vi "Cycle_Diag_Table_Read_Mio.vi"(7 "ERD Data In":T2[](array[typedef]) {"ERD Number" format="%.0x"}, 11 "error in (no error)":errorcluster) -> (2 "Cycle Buffer Status":T1, 3 "Diag Cycle String Out":string[][](array[string]), 15 "error out (no error)":errorcluster)   [LabVIEW 2021]
uses:
  Common/LabVIEW GEA2 Toolkit/GEA3/type defs/ERD Read Data Out.ctl
  type defs/Cycle_Diag_Buffer_Status.ctl
panel:
  out "length":i32
  out "Data":string
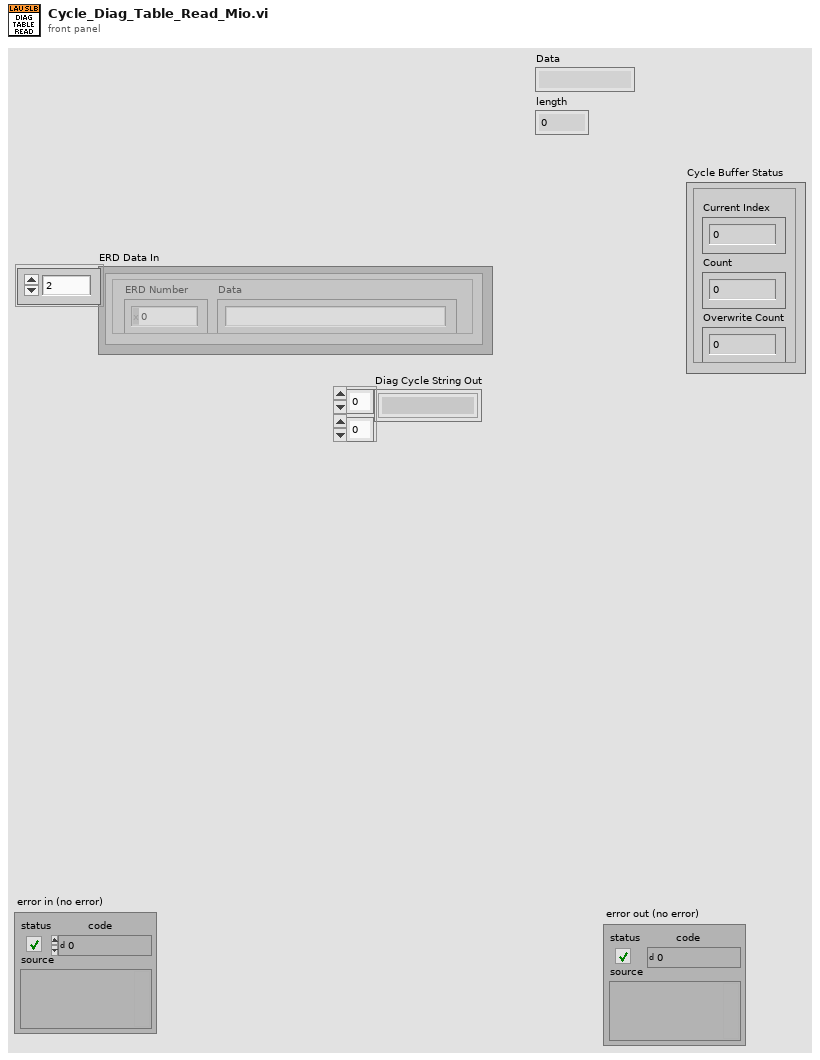
[diagram p1: front panel]
types:
  T1 = typedef "Cycle_Diag_Buffer_Status.ctl" = cluster{"Current Index":u16, "Count":u16, "Overwrite Count":u16}
  T2 = typedef "ERD Read Data Out.ctl" = cluster{"ERD Number":u16, "Data":string}
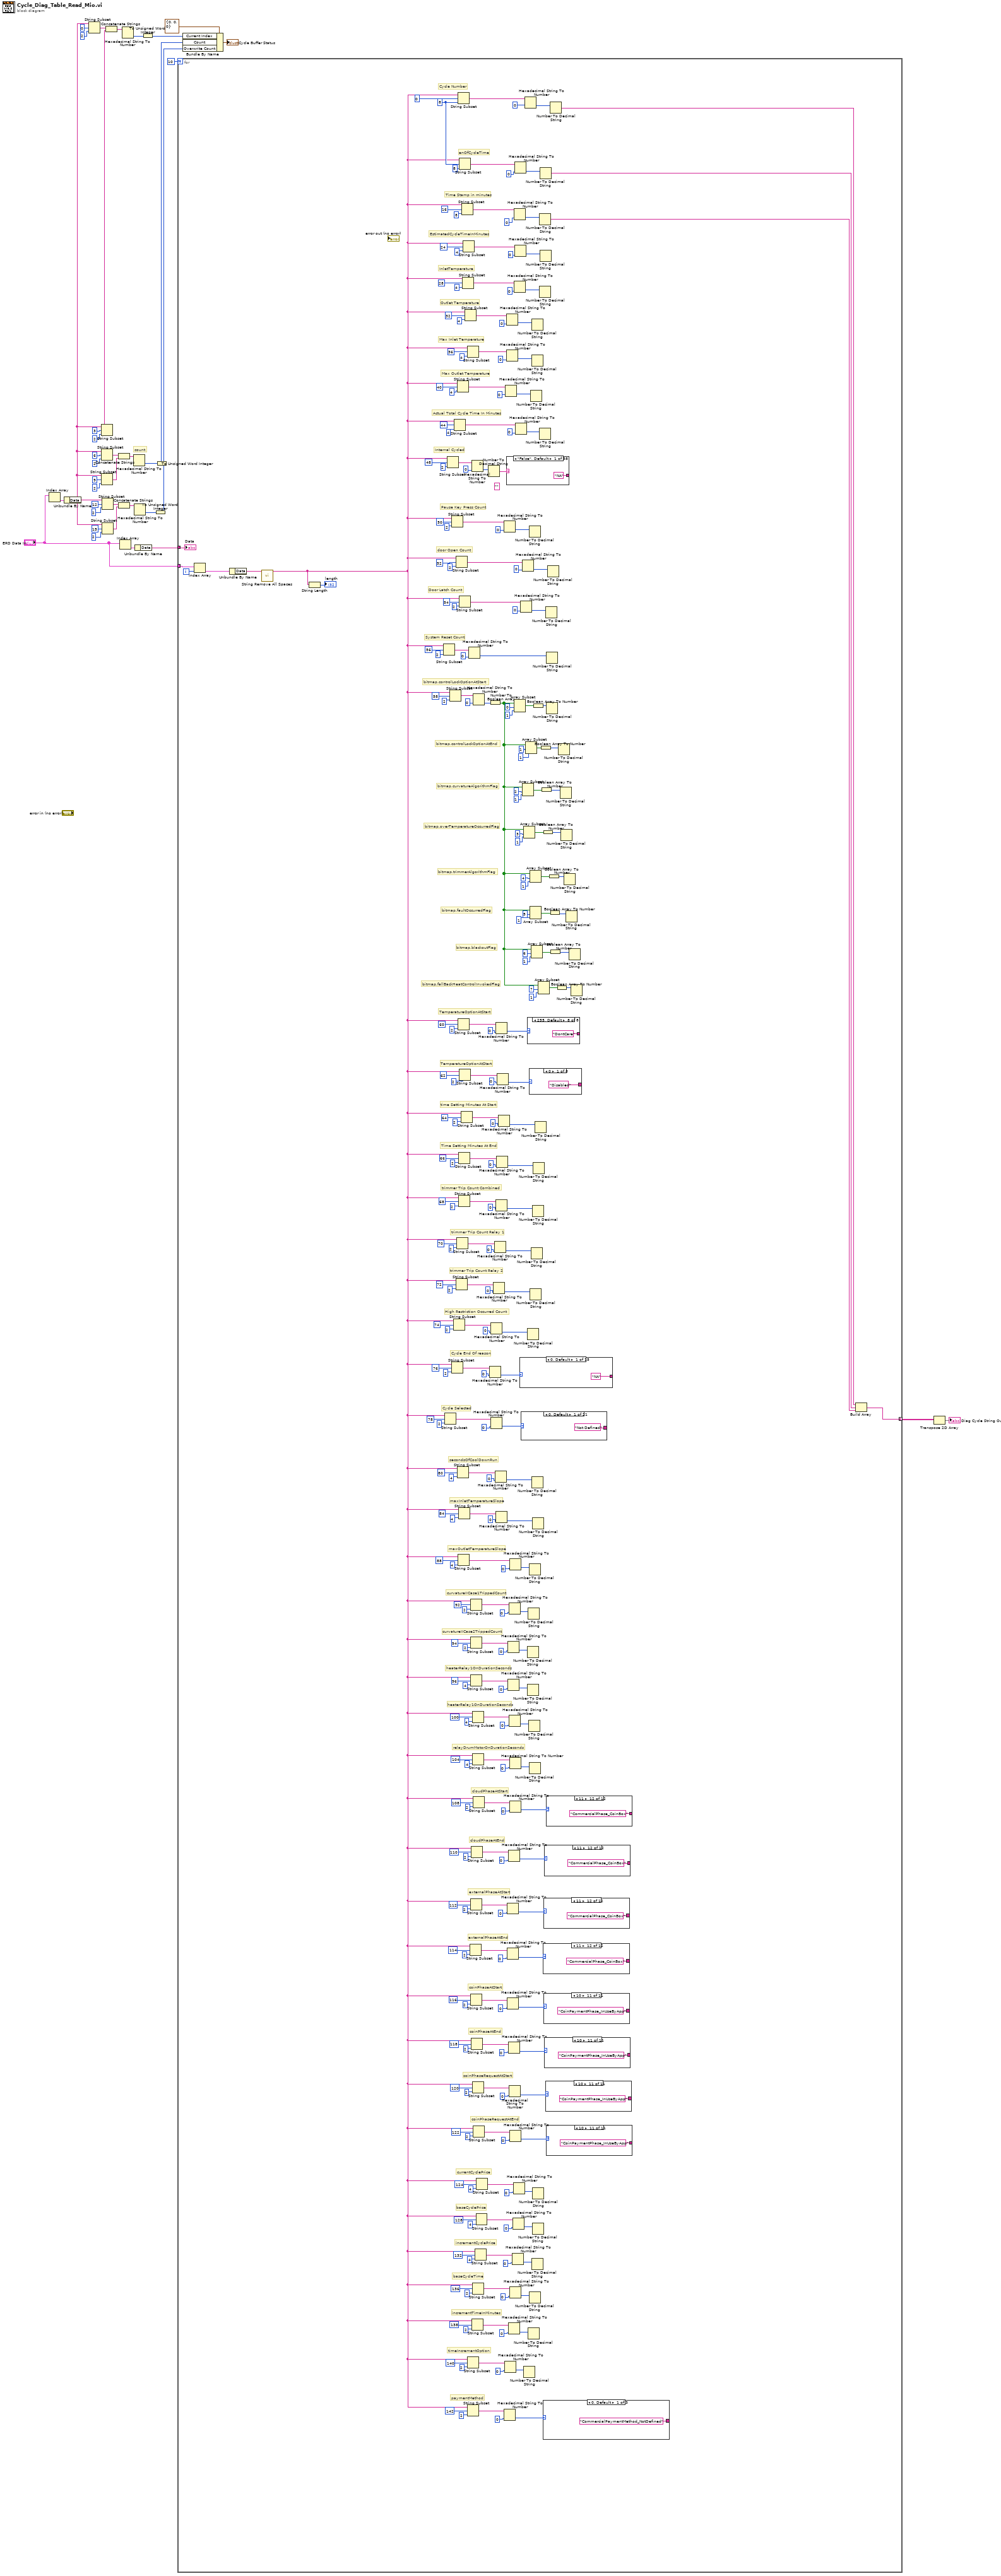
[diagram p0: block diagram]
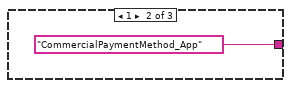
[diagram p2: hidden frame]
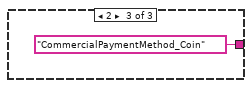
[diagram p3: hidden frame]
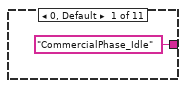
[diagram p4: hidden frame]
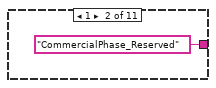
[diagram p5: hidden frame]
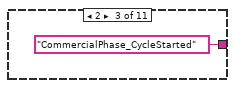
[diagram p6: hidden frame]
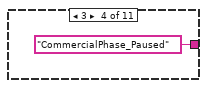
[diagram p7: hidden frame]
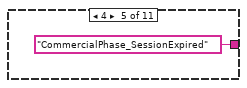
[diagram p8: hidden frame]
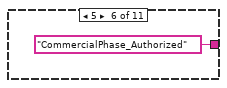
[diagram p9: hidden frame]
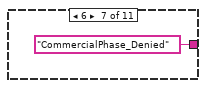
[diagram p10: hidden frame]
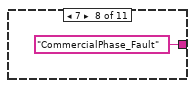
[diagram p11: hidden frame]
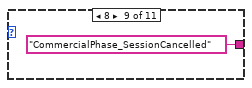
[diagram p12: hidden frame]
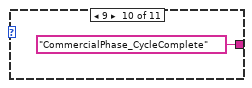
[diagram p13: hidden frame]
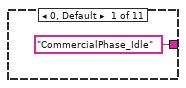
[diagram p14: hidden frame]
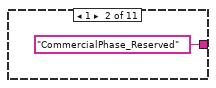
[diagram p15: hidden frame]
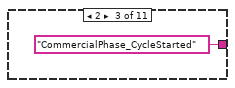
[diagram p16: hidden frame]
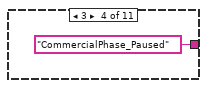
[diagram p17: hidden frame]
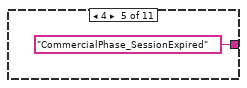
[diagram p18: hidden frame]
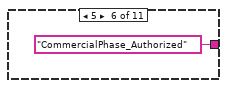
[diagram p19: hidden frame]
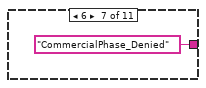
[diagram p20: hidden frame]
diagram:
  # "count"
  n1 = Index Array(array="ERD Data In") -> (element=w30:T2)  [unwired: 1 in]
  n2 = Unbundle By Name(w30) -> ("Data"=w10:string)
  n3 = String Subset(string=w10, offset (0)=0, length (rest)=2 ("length (rest)")) -> (substring=w19:string)
  n4 = String Subset(string=w10, offset (0)=3, length (rest)=2 ("length (rest)")) -> (substring=w20:string)
  n5 = String Subset(string=w10, offset (0)=6, length (rest)=2 ("length (rest)")) -> (substring=w34:string)
  n6 = String Subset(string=w10, offset (0)=9, length (rest)=2 ("length (rest)")) -> (substring=w33:string)
  n7 = String Subset(string=w10, offset (0)=12, length (rest)=2 ("length (rest)")) -> (substring=w21:string)
  n8 = String Subset(string=w10, offset (0)=15, length (rest)=2 ("length (rest)")) -> (substring=w22:string)
  n9 = Concatenate Strings(w19, w20) -> (w23:string)
  n10 = Concatenate Strings(w34, w33) -> (w32:string)
  n11 = Concatenate Strings(w21, w22) -> (w24:string)
  n12 = Index Array(array="ERD Data In") -> (element=w5:T2)  [unwired: 1 in]
  n13 = Hexadecimal String To Number(string=w23) -> (number=w25:u32)  [unwired: 2 in, 1 out]
  n14 = Hexadecimal String To Number(string=w32) -> (number=w31:u32)  [unwired: 2 in, 1 out]
  n15 = Hexadecimal String To Number(string=w24) -> (number=w26:u32)  [unwired: 2 in, 1 out]
  n16 = Unbundle By Name(w5) -> ("Data"=w4:string)
  n17 = To Unsigned Word Integer(number=w25) -> (unsigned 16bit integer=w27:u16)
  n18 = To Unsigned Word Integer(number=w26) -> (unsigned 16bit integer=w28:u16)
  n19 = To Unsigned Word Integer(number=w31) -> (unsigned 16bit integer=w2:u16)
  n20 = for {
    N: 10 -> [_]
    tunnel: [w48] -> w7 mode=indexing
    tunnel: w4 -> [w42]
    tunnel: "ERD Data In" -> [w44]
    i -> [w43]
    (unwired) ""
    w261 = 8 ("length (rest)")
    # "paymentMethod"
    # "timeIncrementOption"
    # "incrementTimeInMinutes"
    # "baseCycleTime"
    # "incrementCyclePrice"
    # "baseCyclePrice"
    # "currentCyclePrice"
    # "coinPhaseRequestAtEnd"
    # "coinPhaseRequestAtStart"
    # "coinPhaseAtEnd"
    # "coinPhaseAtStart"
    # "externalPhaseAtEnd"
    # "externalPhaseAtStart"
    # "cloudPhaseAtEnd"
    # "cloudPhaseAtStart"
    # "relayDrumMotorOnDurationSeconds"
    # "heaterRelay1OnDurationSeconds"
    # "heaterRelay1OnDurationSeconds"
    # "maxInletTemperatureSlope"
    # "secondsOfCoolDownRun"
    # "Cycle End Of reason"
    # "High Restriction Occurred Count"
    # "trimmer Trip Count Relay 2"
    # "trimmer Trip Count Relay 1"
    # "trimmer Trip Count Combined"
    # "Time Setting Minutes At End"
    # "time Setting Minutes At Start"
    # "TemperatureOptionAtStart"
    # "TemperatureOptionAtStart"
    # "bitmap.overTemperatureOccurredFlag"
    # "bitmap.curvatureAlgorithmFlag"
    # "bitmap.controlLockOptionAtEnd"
    # "Pause Key Press Count"
    # "InletTemperature"
    # "curvatureIICase1TrippedCount"
    # "curvatureIICase2TrippedCount"
    # "maxOutletTemperatureSlope"
    # "Cycle Selected"
    # "bitmap.fallBackHeatControlInvokedFlag"
    # "bitmap.blackoutFlag"
    # "bitmap.faultOccurredFlag"
    # "bitmap.trimmerAlgorithmFlag"
    # "bitmap.controlLockOptionAtStart"
    # "System Reset Count"
    # "Door Latch Count"
    # "door Open Count"
    # "Internal Cycled"
    # "Actual Total Cycle Time In Minutes"
    # "Max Outlet Temperature"
    # "Max Inlet Temperature"
    # "Outlet Temperature"
    # "EstimatedCycleTimeInMinutes"
    # "Time Stamp in minutes"
    # "enOfCycleTime"
    # "Cycle Number"
    n21 = Index Array(array=w44, index=w43) -> (element=w41:T2)
    n22 = Unbundle By Name(w41) -> ("Data"=w39:string)
    n23 = call "String Remove All Spaces.vi"("Input String"=w39) -> ("Spaces Removed"=w38:string)  [unwired: 13 in, 1 out]
    n24 = String Length(string=w38) -> (length=→"length":i32)
    n25 = String Subset(string=w38, offset (0)=56, length (rest)=2 ("length (rest)")) -> (substring=w235:string)
    n26 = String Subset(string=w38, offset (0)=78, length (rest)=2 ("length (rest)")) -> (substring=w272:string)
    n27 = String Subset(string=w38, offset (0)=48, length (rest)=2 ("length (rest)")) -> (substring=w245:string)
    n28 = String Subset(string=w38, offset (0)=58, length (rest)=2 ("length (rest)")) -> (substring=w234:string)
    n29 = String Subset(string=w38, offset (0)=50, length (rest)=2 ("length (rest)")) -> (substring=w242:string)
    n30 = String Subset(string=w38, offset (0)=76, length (rest)=2 ("length (rest)")) -> (substring=w192:string)
    n31 = String Subset(string=w38, offset (0)=74, length (rest)=2 ("length (rest)")) -> (substring=w193:string)
    n32 = String Subset(string=w38, offset (0)=44, length (rest)=4 ("length (rest)")) -> (substring=w247:string)
    n33 = String Subset(string=w38, offset (0)=72, length (rest)=2 ("length (rest)")) -> (substring=w200:string)
    n34 = String Subset(string=w38, offset (0)=52, length (rest)=2 ("length (rest)")) -> (substring=w240:string)
    n35 = String Subset(string=w38, offset (0)=70, length (rest)=2 ("length (rest)")) -> (substring=w205:string)
    n36 = String Subset(string=w38, offset (0)=40, length (rest)=4 ("length (rest)")) -> (substring=w249:string)
    n37 = String Subset(string=w38, offset (0)=80, length (rest)=4 ("length (rest)")) -> (substring=w181:string)
    n38 = String Subset(string=w38, offset (0)=0, length (rest)=w261) -> (substring=w262:string)
    n39 = String Subset(string=w38, offset (0)=60, length (rest)=2 ("length (rest)")) -> (substring=w231:string)
    n40 = String Subset(string=w38, offset (0)=88, length (rest)=4 ("length (rest)")) -> (substring=w269:string)
    n41 = String Subset(string=w38, offset (0)=68, length (rest)=2 ("length (rest)")) -> (substring=w210:string)
    n42 = String Subset(string=w38, offset (0)=84, length (rest)=4 ("length (rest)")) -> (substring=w180:string)
    n43 = String Subset(string=w38, offset (0)=66, length (rest)=2 ("length (rest)")) -> (substring=w215:string)
    n44 = String Subset(string=w38, offset (0)=w261, length (rest)=8 ("length (rest)")) -> (substring=w260:string)
    n45 = String Subset(string=w38, offset (0)=54, length (rest)=2 ("length (rest)")) -> (substring=w238:string)
    n46 = String Subset(string=w38, offset (0)=62, length (rest)=2 ("length (rest)")) -> (substring=w224:string)
    n47 = String Subset(string=w38, offset (0)=64, length (rest)=2 ("length (rest)")) -> (substring=w220:string)
    n48 = String Subset(string=w38, offset (0)=16, length (rest)=8 ("length (rest)")) -> (substring=w259:string)
    n49 = String Subset(string=w38, offset (0)=28, length (rest)=4 ("length (rest)")) -> (substring=w255:string)
    n50 = String Subset(string=w38, offset (0)=24, length (rest)=4 ("length (rest)")) -> (substring=w257:string)
    n51 = String Subset(string=w38, offset (0)=32, length (rest)=4 ("length (rest)")) -> (substring=w253:string)
    n52 = String Subset(string=w38, offset (0)=36, length (rest)=4 ("length (rest)")) -> (substring=w251:string)
    n53 = String Subset(string=w38, offset (0)=142, length (rest)=2 ("length (rest)")) -> (substring=w85:string)
    n54 = String Subset(string=w38, offset (0)=140, length (rest)=2 ("length (rest)")) -> (substring=w89:string)
    n55 = Hexadecimal String To Number(string=w235, default (0uL)=u16 0) -> (number=w276:u16)  [unwired: 1 in, 1 out]
    n56 = String Subset(string=w38, offset (0)=114, length (rest)=2 ("length (rest)")) -> (substring=w140:string)
    n57 = String Subset(string=w38, offset (0)=92, length (rest)=2 ("length (rest)")) -> (substring=w266:string)
    n58 = String Subset(string=w38, offset (0)=112, length (rest)=2 ("length (rest)")) -> (substring=w145:string)
    n59 = String Subset(string=w38, offset (0)=116, length (rest)=2 ("length (rest)")) -> (substring=w135:string)
    n60 = String Subset(string=w38, offset (0)=94, length (rest)=2 ("length (rest)")) -> (substring=w263:string)
    n61 = String Subset(string=w38, offset (0)=96, length (rest)=4 ("length (rest)")) -> (substring=w171:string)
    n62 = String Subset(string=w38, offset (0)=110, length (rest)=2 ("length (rest)")) -> (substring=w150:string)
    n63 = String Subset(string=w38, offset (0)=118, length (rest)=2 ("length (rest)")) -> (substring=w130:string)
    n64 = Hexadecimal String To Number(string=w245, default (0uL)=u32 0) -> (number=w284:u32)  [unwired: 1 in, 1 out]
    n65 = String Subset(string=w38, offset (0)=138, length (rest)=2 ("length (rest)")) -> (substring=w94:string)
    n66 = String Subset(string=w38, offset (0)=100, length (rest)=4 ("length (rest)")) -> (substring=w164:string)
    n67 = String Subset(string=w38, offset (0)=120, length (rest)=2 ("length (rest)")) -> (substring=w120:string)
    n68 = String Subset(string=w38, offset (0)=104, length (rest)=4 ("length (rest)")) -> (substring=w161:string)
    n69 = String Subset(string=w38, offset (0)=136, length (rest)=2 ("length (rest)")) -> (substring=w101:string)
    n70 = Hexadecimal String To Number(string=w234, default (0uL)=u16 0) -> (number=w79:u16)  [unwired: 1 in, 1 out]
    n71 = String Subset(string=w38, offset (0)=108, length (rest)=2 ("length (rest)")) -> (substring=w155:string)
    n72 = String Subset(string=w38, offset (0)=122, length (rest)=2 ("length (rest)")) -> (substring=w125:string)
    n73 = String Subset(string=w38, offset (0)=132, length (rest)=4 ("length (rest)")) -> (substring=w106:string)
    n74 = String Subset(string=w38, offset (0)=128, length (rest)=4 ("length (rest)")) -> (substring=w109:string)
    n75 = String Subset(string=w38, offset (0)=124, length (rest)=4 ("length (rest)")) -> (substring=w116:string)
    n76 = Number To Decimal String(number=w284) -> (decimal integer string=w243:string)  [unwired: 1 in]
    n77 = Hexadecimal String To Number(string=w192, default (0uL)=u8 0) -> (number=w188:u8)  [unwired: 1 in, 1 out]
    n78 = Number To Boolean Array(number=w79) -> (Boolean array=w49:bool[])
    n79 = Hexadecimal String To Number(string=w272, default (0uL)=u32 0) -> (number=w186:u32)  [unwired: 1 in, 1 out]
    n80 = Hexadecimal String To Number(string=w193, default (0uL)=u32 0) -> (number=w197:u32)  [unwired: 1 in, 1 out]
    n81 = Hexadecimal String To Number(string=w200, default (0uL)=u8 0) -> (number=w198:u8)  [unwired: 1 in, 1 out]
    n82 = Hexadecimal String To Number(string=w205, default (0uL)=u32 0) -> (number=w207:u32)  [unwired: 1 in, 1 out]
    n83 = Hexadecimal String To Number(string=w181, default (0uL)=u32 0) -> (number=w185:u32)  [unwired: 1 in, 1 out]
    n84 = Hexadecimal String To Number(string=w231, default (0uL)=u32 0) -> (number=w228:u32)  [unwired: 1 in, 1 out]
    n85 = Hexadecimal String To Number(string=w210, default (0uL)=u32 0) -> (number=w208:u32)  [unwired: 1 in, 1 out]
    n86 = Hexadecimal String To Number(string=w180, default (0uL)=u8 0) -> (number=w176:u8)  [unwired: 1 in, 1 out]
    n87 = Hexadecimal String To Number(string=w215, default (0uL)=u32 0) -> (number=w217:u32)  [unwired: 1 in, 1 out]
    n88 = Hexadecimal String To Number(string=w224, default (0uL)=u32 0) -> (number=w227:u32)  [unwired: 1 in, 1 out]
    n89 = Hexadecimal String To Number(string=w220, default (0uL)=u32 0) -> (number=w218:u32)  [unwired: 1 in, 1 out]
    n90 = Hexadecimal String To Number(string=w242, default (0uL)=u16 0) -> (number=w281:u16)  [unwired: 1 in, 1 out]
    n91 = Hexadecimal String To Number(string=w85, default (0uL)=u8 0) -> (number=w83:u8)  [unwired: 1 in, 1 out]
    n92 = Hexadecimal String To Number(string=w89, default (0uL)=u8 0) -> (number=w90:u8)  [unwired: 1 in, 1 out]
    n93 = Hexadecimal String To Number(string=w249, default (0uL)=u32 0) -> (number=w288:u32)  [unwired: 1 in, 1 out]
    n94 = Hexadecimal String To Number(string=w253, default (0uL)=u32 0) -> (number=w292:u32)  [unwired: 1 in, 1 out]
    n95 = Hexadecimal String To Number(string=w251, default (0uL)=u32 0) -> (number=w289:u32)  [unwired: 1 in, 1 out]
    n96 = case shown="\"False\", Default" w243 {
      tunnel: ["NA" "Unmapped" "MixedLoad" "Casuals" "Delicates" "SpeedDry" "Jeans" "TimedDry" "WarmUp" "AirFluff" "SteamDewrinkle" "SteamRefresh" "SanitizeDry" "BulkyItems" "TowelsSheets" "Cottons" "CasualsLessDry" "CasualsMoreDry" "CottonsLessDry" "CottonsOptimumDry" "CottonsMoreDry" "DelicatesLessDry" "DelicatesMoreDry" "TimedDry1" "TimedDry2" "TimedDry3" "TimedDry4" "TimedDry5" "TimedDry6" "ActiveWear" "DeWrinkle" "EnergySaver" "WasherLink" "BlockedVent" "SmartVent" "Scent" "Max" "Downloaded"] -> _
      frame "False", Default {
      }
      frame "0" {
      }
      frame "1" {
      }
      frame "2" {
      }
      frame "3" {
      }
      frame "4" {
      }
      frame "5" {
      }
      frame "6" {
      }
      frame "7" {
      }
      frame "8" {
      }
      frame "9" {
      }
      frame "10" {
      }
      frame "11" {
      }
      frame "12" {
      }
      frame "13" {
      }
      frame "14" {
      }
      frame "15" {
      }
      frame "16" {
      }
      frame "17" {
      }
      frame "18" {
      }
      frame "19" {
      }
      frame "20" {
      }
      frame "21" {
      }
      frame "22" {
      }
      frame "23" {
      }
      frame "24" {
      }
      frame "25" {
      }
      frame "26" {
      }
      frame "27" {
      }
      frame "28" {
      }
      frame "29" {
      }
      frame "30" {
      }
      frame "31" {
      }
      frame "32" {
      }
      frame "33" {
      }
      frame "34" {
      }
      frame "35" {
      }
      frame "36" {
      }
    }
    n97 = Hexadecimal String To Number(string=w140, default (0uL)=u8 0) -> (number=w142:u8)  [unwired: 1 in, 1 out]
    n98 = Hexadecimal String To Number(string=w145, default (0uL)=u8 0) -> (number=w143:u8)  [unwired: 1 in, 1 out]
    n99 = Hexadecimal String To Number(string=w135, default (0uL)=u8 0) -> (number=w133:u8)  [unwired: 1 in, 1 out]
    n100 = Hexadecimal String To Number(string=w263, default (0uL)=u32 0) -> (number=w264:u32)  [unwired: 1 in, 1 out]
    n101 = Hexadecimal String To Number(string=w171, default (0uL)=u32 0) -> (number=w170:u32)  [unwired: 1 in, 1 out]
    n102 = Hexadecimal String To Number(string=w150, default (0uL)=u8 0) -> (number=w152:u8)  [unwired: 1 in, 1 out]
    n103 = Hexadecimal String To Number(string=w130, default (0uL)=u8 0) -> (number=w132:u8)  [unwired: 1 in, 1 out]
    n104 = Hexadecimal String To Number(string=w94, default (0uL)=u32 0) -> (number=w95:u32)  [unwired: 1 in, 1 out]
    n105 = Hexadecimal String To Number(string=w266, default (0uL)=u32 0) -> (number=w268:u32)  [unwired: 1 in, 1 out]
    n106 = Hexadecimal String To Number(string=w164, default (0uL)=u32 0) -> (number=w165:u32)  [unwired: 1 in, 1 out]
    n107 = Hexadecimal String To Number(string=w120, default (0uL)=u8 0) -> (number=w122:u8)  [unwired: 1 in, 1 out]
    n108 = Hexadecimal String To Number(string=w161, default (0uL)=u32 0) -> (number=w160:u32)  [unwired: 1 in, 1 out]
    n109 = Hexadecimal String To Number(string=w101, default (0uL)=u8 0) -> (number=w100:u8)  [unwired: 1 in, 1 out]
    n110 = Hexadecimal String To Number(string=w269, default (0uL)=u32 0) -> (number=w270:u32)  [unwired: 1 in, 1 out]
    n111 = Hexadecimal String To Number(string=w155, default (0uL)=u8 0) -> (number=w153:u8)  [unwired: 1 in, 1 out]
    n112 = Hexadecimal String To Number(string=w125, default (0uL)=u8 0) -> (number=w123:u8)  [unwired: 1 in, 1 out]
    n113 = Hexadecimal String To Number(string=w106, default (0uL)=u32 0) -> (number=w105:u32)  [unwired: 1 in, 1 out]
    n114 = Hexadecimal String To Number(string=w109, default (0uL)=u32 0) -> (number=w110:u32)  [unwired: 1 in, 1 out]
    n115 = Hexadecimal String To Number(string=w116, default (0uL)=u32 0) -> (number=w115:u32)  [unwired: 1 in, 1 out]
    n116 = Array Subset(array=w49, index=0, length=1) -> (w80:bool[])
    n117 = Hexadecimal String To Number(string=w259, default (0uL)=u32 0) -> (number=w300:u32)  [unwired: 1 in, 1 out]
    n118 = Hexadecimal String To Number(string=w255, default (0uL)=u32 0) -> (number=w293:u32)  [unwired: 1 in, 1 out]
    n119 = Hexadecimal String To Number(string=w260, default (0uL)=u32 0) -> (number=w301:u32)  [unwired: 1 in, 1 out]
    n120 = Hexadecimal String To Number(string=w257, default (0uL)=u32 0) -> (number=w299:u32)  [unwired: 1 in, 1 out]
    n121 = Hexadecimal String To Number(string=w247, default (0uL)=u32 0) -> (number=w285:u32)  [unwired: 1 in, 1 out]
    n122 = case shown="0, Default" w188 {
      tunnel: ["NA" "EmptyDrum" "DryLoad" "CoolDownPaused" "xtendedTumblePaused" "KnobChange" "PowerButtonPressed" "CycleComplete" "EventSequenceCommunicationIssue" "CriticalFault" "RemoteStop" "ExtremeHeatDetected" "NonPausableCyclePaused" "SafetyCriticalWatchdogTimeout" "DontCare"] -> _
      frame 0, Default {
      }
      frame 1 {
      }
      frame 2 {
      }
      frame 3 {
      }
      frame 4 {
      }
      frame 5 {
      }
      frame 6 {
      }
      frame 7 {
      }
      frame 8 {
      }
      frame 9 {
      }
      frame 10 {
      }
      frame 11 {
      }
      frame 12 {
      }
      frame 13 {
      }
      frame 14 {
      }
    }
    n123 = Hexadecimal String To Number(string=w238, default (0uL)=u16 0) -> (number=w277:u16)  [unwired: 1 in, 1 out]
    n124 = case shown="0, Default" w186 {
      tunnel: ["Not Defined" "Bulky Items" "Sanitize" "Towels/Sheets" "Mixed Load" "Jeans" "Delicates" "Cottons" "Easy Care" "Active Wear" "Timed Dry" "DeWrinkle" "Quick/Air Fluff" "Steam Refresh" "Steam Dewrinkle" "Speed Dry" "Mixed" "Quick dry" "Casuals" "Warm up" "Energy Saver"] -> _
      frame 0, Default {
      }
      frame 4 {
      }
      frame 5 {
      }
      frame 6 {
      }
      frame 8 {
      }
      frame 11 {
      }
      frame 13 {
      }
      frame 128 {
      }
      frame 129 {
      }
      frame 130 {
      }
      frame 131 {
      }
      frame 132 {
      }
      frame 133 {
      }
      frame 134 {
      }
      frame 135 {
      }
      frame 136 {
      }
      frame 137 {
      }
      frame 138 {
      }
      frame 139 {
      }
      frame 140 {
      }
      frame 141 {
      }
    }
    n125 = Hexadecimal String To Number(string=w240, default (0uL)=u16 0) -> (number=w280:u16)  [unwired: 1 in, 1 out]
    n126 = Array Subset(array=w49, index=2, length=1) -> (w71:bool[])
    n127 = Array Subset(array=w49, index=3, length=1) -> (w67:bool[])
    n128 = Number To Decimal String(number=w90) -> ()  [unwired: 1 in, 1 out]
    n129 = Hexadecimal String To Number(string=w262, default (0uL)=u32 0) -> (number=w302:u32)  [unwired: 1 in, 1 out]
    n130 = Array Subset(array=w49, index=1, length=1) -> (w75:bool[])
    n131 = Number To Decimal String(number=w264) -> ()  [unwired: 1 in, 1 out]
    n132 = Number To Decimal String(number=w170) -> ()  [unwired: 1 in, 1 out]
    n133 = case shown="255, Default" w228 {
      tunnel: ["Disabled" "NoHeat" "ExtraLow" "Low" "Medium" "High" "Max" "DontCare"] -> _
      frame 0 {
      }
      frame 1 {
      }
      frame 2 {
      }
      frame 3 {
      }
      frame 4 {
      }
      frame 5 {
      }
      frame 6 {
      }
      frame 255, Default {
      }
    }
    n134 = Number To Decimal String(number=w197) -> ()  [unwired: 1 in, 1 out]
    n135 = Number To Decimal String(number=w95) -> ()  [unwired: 1 in, 1 out]
    n136 = Number To Decimal String(number=w268) -> ()  [unwired: 1 in, 1 out]
    n137 = Number To Decimal String(number=w165) -> ()  [unwired: 1 in, 1 out]
    n138 = Number To Decimal String(number=w281) -> ()  [unwired: 1 in, 1 out]
    n139 = case shown="0" w227 {
      tunnel: ["Disabled" "NoHeat" "ExtraLow" "Low" "Medium" "High" "Max" "DontCare"] -> _
      frame 0 {
      }
      frame 1 {
      }
      frame 2 {
      }
      frame 3 {
      }
      frame 4 {
      }
      frame 5 {
      }
      frame 6 {
      }
      frame 255, Default {
      }
    }
    n140 = Number To Decimal String(number=w160) -> ()  [unwired: 1 in, 1 out]
    n141 = Number To Decimal String(number=w100) -> ()  [unwired: 1 in, 1 out]
    n142 = Number To Decimal String(number=w270) -> ()  [unwired: 1 in, 1 out]
    n143 = Array Subset(array=w49, index=4, length=1) -> (w63:bool[])
    n144 = Array Subset(array=w49, index=5, length=1) -> (w59:bool[])
    n145 = Number To Decimal String(number=w198) -> ()  [unwired: 1 in, 1 out]
    n146 = Number To Decimal String(number=w288) -> ()  [unwired: 1 in, 1 out]
    n147 = Array Subset(array=w49, index=6, length=1) -> (w55:bool[])
    n148 = Number To Decimal String(number=w207) -> ()  [unwired: 1 in, 1 out]
    n149 = Number To Decimal String(number=w292) -> ()  [unwired: 1 in, 1 out]
    n150 = Number To Decimal String(number=w289) -> ()  [unwired: 1 in, 1 out]
    n151 = Number To Decimal String(number=w185) -> ()  [unwired: 1 in, 1 out]
    n152 = Number To Decimal String(number=w105) -> ()  [unwired: 1 in, 1 out]
    n153 = Number To Decimal String(number=w110) -> ()  [unwired: 1 in, 1 out]
    n154 = Boolean Array To Number(Boolean array=w80) -> (number=w78:u32)
    n155 = Number To Decimal String(number=w208) -> ()  [unwired: 1 in, 1 out]
    n156 = Number To Decimal String(number=w176) -> ()  [unwired: 1 in, 1 out]
    n157 = Number To Decimal String(number=w115) -> ()  [unwired: 1 in, 1 out]
    n158 = Number To Decimal String(number=w217) -> ()  [unwired: 1 in, 1 out]
    n159 = Number To Decimal String(number=w218) -> ()  [unwired: 1 in, 1 out]
    n160 = Array Subset(array=w49, index=7, length=1) -> (w51:bool[])
    n161 = Number To Decimal String(number=w300) -> (decimal integer string=w45:string)  [unwired: 1 in]
    n162 = Number To Decimal String(number=w293) -> ()  [unwired: 1 in, 1 out]
    n163 = Number To Decimal String(number=w285) -> ()  [unwired: 1 in, 1 out]
    n164 = Number To Decimal String(number=w301) -> (decimal integer string=w46:string)  [unwired: 1 in]
    n165 = Number To Decimal String(number=w299) -> ()  [unwired: 1 in, 1 out]
    n166 = Boolean Array To Number(Boolean array=w75) -> (number=w74:u32)
    n167 = Boolean Array To Number(Boolean array=w71) -> (number=w70:u32)
    n168 = Boolean Array To Number(Boolean array=w67) -> (number=w66:u32)
    n169 = case shown="0, Default" w83 {
      tunnel: ["CommercialPaymentMethod_NotDefined" "CommercialPaymentMethod_App" "CommercialPaymentMethod_Coin"] -> _
      frame 0, Default {
      }
      frame 1 {
      }
      frame 2 {
      }
    }
    n170 = case shown="11" w142 {
      tunnel: ["CommercialPhase_Idle" "CommercialPhase_Reserved" "CommercialPhase_CycleRequested" "CommercialPhase_CycleStarted" "CommercialPhase_Paused" "CommercialPhase_SessionExpired" "CommercialPhase_Authorized" "CommercialPhase_Denied" "CommercialPhase_Fault" "CommercialPhase_SessionCancelled" "CommercialPhase_CycleComplete" "CommercialPhase_CoinBox"] -> _
      frame 0, Default {
      }
      frame 1 {
      }
      frame 2 {
      }
      frame 3 {
      }
      frame 4 {
      }
      frame 5 {
      }
      frame 6 {
      }
      frame 7 {
      }
      frame 8 {
      }
      frame 9 {
      }
      frame 10 {
      }
      frame 11 {
      }
    }
    n171 = case shown="11" w143 {
      tunnel: ["CommercialPhase_Idle" "CommercialPhase_Reserved" "CommercialPhase_CycleRequested" "CommercialPhase_CycleStarted" "CommercialPhase_Paused" "CommercialPhase_SessionExpired" "CommercialPhase_Authorized" "CommercialPhase_Denied" "CommercialPhase_Fault" "CommercialPhase_SessionCancelled" "CommercialPhase_CycleComplete" "CommercialPhase_CoinBox"] -> _
      frame 0, Default {
      }
      frame 1 {
      }
      frame 2 {
      }
      frame 3 {
      }
      frame 4 {
      }
      frame 5 {
      }
      frame 6 {
      }
      frame 7 {
      }
      frame 8 {
      }
      frame 9 {
      }
      frame 10 {
      }
      frame 11 {
      }
    }
    n172 = case shown="10" w133 {
      tunnel: ["CommercialPhase_Idle" "CommercialPhase_Reserved" "CommercialPhase_CycleStarted" "CommercialPhase_Paused" "CommercialPhase_SessionExpired" "CommercialPhase_Authorized" "CommercialPhase_Denied" "CommercialPhase_Fault" "CommercialPhase_SessionCancelled" "CommercialPhase_CycleComplete" "CoinPaymentPhase_InUseByApp"] -> _
      frame 0, Default {
      }
      frame 1 {
      }
      frame 2 {
      }
      frame 3 {
      }
      frame 4 {
      }
      frame 5 {
      }
      frame 6 {
      }
      frame 7 {
      }
      frame 8 {
      }
      frame 9 {
      }
      frame 10 {
      }
    }
    n173 = case shown="11" w152 {
      tunnel: ["CommercialPhase_Idle" "CommercialPhase_Reserved" "CommercialPhase_CycleRequested" "CommercialPhase_CycleStarted" "CommercialPhase_Paused" "CommercialPhase_SessionExpired" "CommercialPhase_Authorized" "CommercialPhase_Denied" "CommercialPhase_Fault" "CommercialPhase_SessionCancelled" "CommercialPhase_CycleComplete" "CommercialPhase_CoinBox"] -> _
      frame 0, Default {
      }
      frame 1 {
      }
      frame 2 {
      }
      frame 3 {
      }
      frame 4 {
      }
      frame 5 {
      }
      frame 6 {
      }
      frame 7 {
      }
      frame 8 {
      }
      frame 9 {
      }
      frame 10 {
      }
      frame 11 {
      }
    }
    n174 = case shown="10" w132 {
      tunnel: ["CommercialPhase_Idle" "CommercialPhase_Reserved" "CommercialPhase_CycleStarted" "CommercialPhase_Paused" "CommercialPhase_SessionExpired" "CommercialPhase_Authorized" "CommercialPhase_Denied" "CommercialPhase_Fault" "CommercialPhase_SessionCancelled" "CommercialPhase_CycleComplete" "CoinPaymentPhase_InUseByApp"] -> _
      frame 0, Default {
      }
      frame 1 {
      }
      frame 2 {
      }
      frame 3 {
      }
      frame 4 {
      }
      frame 5 {
      }
      frame 6 {
      }
      frame 7 {
      }
      frame 8 {
      }
      frame 9 {
      }
      frame 10 {
      }
    }
    n175 = case shown="10" w122 {
      tunnel: ["CommercialPhase_Idle" "CommercialPhase_Reserved" "CommercialPhase_CycleStarted" "CommercialPhase_Paused" "CommercialPhase_SessionExpired" "CommercialPhase_Authorized" "CommercialPhase_Denied" "CommercialPhase_Fault" "CommercialPhase_SessionCancelled" "CommercialPhase_CycleComplete" "CoinPaymentPhase_InUseByApp"] -> _
      frame 0, Default {
      }
      frame 1 {
      }
      frame 2 {
      }
      frame 3 {
      }
      frame 4 {
      }
      frame 5 {
      }
      frame 6 {
      }
      frame 7 {
      }
      frame 8 {
      }
      frame 9 {
      }
      frame 10 {
      }
    }
    n176 = Number To Decimal String(number=w277) -> ()  [unwired: 1 in, 1 out]
    n177 = case shown="11" w153 {
      tunnel: ["CommercialPhase_Idle" "CommercialPhase_Reserved" "CommercialPhase_CycleRequested" "CommercialPhase_CycleStarted" "CommercialPhase_Paused" "CommercialPhase_SessionExpired" "CommercialPhase_Authorized" "CommercialPhase_Denied" "CommercialPhase_Fault" "CommercialPhase_SessionCancelled" "CommercialPhase_CycleComplete" "CommercialPhase_CoinBox"] -> _
      frame 0, Default {
      }
      frame 1 {
      }
      frame 2 {
      }
      frame 3 {
      }
      frame 4 {
      }
      frame 5 {
      }
      frame 6 {
      }
      frame 7 {
      }
      frame 8 {
      }
      frame 9 {
      }
      frame 10 {
      }
      frame 11 {
      }
    }
    n178 = case shown="10" w123 {
      tunnel: ["CommercialPhase_Idle" "CommercialPhase_Reserved" "CommercialPhase_CycleStarted" "CommercialPhase_Paused" "CommercialPhase_SessionExpired" "CommercialPhase_Authorized" "CommercialPhase_Denied" "CommercialPhase_Fault" "CommercialPhase_SessionCancelled" "CommercialPhase_CycleComplete" "CoinPaymentPhase_InUseByApp"] -> _
      frame 0, Default {
      }
      frame 1 {
      }
      frame 2 {
      }
      frame 3 {
      }
      frame 4 {
      }
      frame 5 {
      }
      frame 6 {
      }
      frame 7 {
      }
      frame 8 {
      }
      frame 9 {
      }
      frame 10 {
      }
    }
    n179 = Number To Decimal String(number=w276) -> ()  [unwired: 1 in, 1 out]
    n180 = Number To Decimal String(number=w78) -> ()  [unwired: 1 in, 1 out]
    n181 = Number To Decimal String(number=w280) -> ()  [unwired: 1 in, 1 out]
    n182 = Boolean Array To Number(Boolean array=w63) -> (number=w62:u32)
    n183 = Boolean Array To Number(Boolean array=w59) -> (number=w58:u32)
    n184 = Boolean Array To Number(Boolean array=w55) -> (number=w54:u32)
    n185 = Number To Decimal String(number=w302) -> (decimal integer string=w47:string)  [unwired: 1 in]
    n186 = Boolean Array To Number(Boolean array=w51) -> (number=w50:u32)
    n187 = Number To Decimal String(number=w74) -> ()  [unwired: 1 in, 1 out]
    n188 = Number To Decimal String(number=w70) -> ()  [unwired: 1 in, 1 out]
    n189 = Number To Decimal String(number=w66) -> ()  [unwired: 1 in, 1 out]
    n190 = Number To Decimal String(number=w62) -> ()  [unwired: 1 in, 1 out]
    n191 = Number To Decimal String(number=w58) -> ()  [unwired: 1 in, 1 out]
    n192 = Number To Decimal String(number=w54) -> ()  [unwired: 1 in, 1 out]
    n193 = Number To Decimal String(number=w50) -> ()  [unwired: 1 in, 1 out]
    n194 = Build Array(w47, w46, w45) -> (w48:string[])
    "Data" <- w42
  }
  n195 = Bundle By Name(cluster=T1 {"Current Index"=0, "Count"=0, "Overwrite Count"=0} ("Cycle Buffer Status"), "Current Index"=w27, "Count"=w2, "Overwrite Count"=w28) -> (→"Cycle Buffer Status":T1)
  n196 = Transpose 2D Array(2D array=w7) -> (transposed array=→"Diag Cycle String Out":string[][])
